vi "Konvolucio MUDS150628 CP1540 Tool.vi"() -> ()   [LabVIEW 2011]
uses:
  <instrlib>/Konvolucio MUDS150628/Types/DtcItemType.ctl
  <vilib>/Utility/miscctls.llb/LVRowAndColumnUnsignedTypeDef.ctl
  <instrlib>/Konvolucio MUDS150628/Types/UdsHandleType.ctl
  <instrlib>/Konvolucio MCAN120803/Types/MCanHandleType.ctl
  <instrlib>/Konvolucio MUDS150628/Public/Low CAN/Attributes/AttrGetPendingMsg.vi
  <instrlib>/Konvolucio MUDS150628/Public/Low CAN/Attributes/AttrGetRxTotal.vi
  <instrlib>/Konvolucio MUDS150628/Public/Low CAN/Attributes/AttrGetRxErrorCounter.vi
  <instrlib>/Konvolucio MUDS150628/Public/Low CAN/Attributes/AttrGetRxDrop.vi
  <instrlib>/Konvolucio MUDS150628/Public/Low CAN/Attributes/AttrGetTxTotal.vi
  <instrlib>/Konvolucio MUDS150628/Public/Low CAN/Attributes/AttrGetTxErrorCounter.vi
  <instrlib>/Konvolucio MUDS150628/Public/Low CAN/Attributes/AttrGetTxDrop.vi
  <instrlib>/Konvolucio MUDS150628/Public/Low CAN/Attributes/AttrSetTermination.vi
  <instrlib>/Konvolucio MUDS150628/Public/Low CAN/Attributes/AttrGetFirmwareRev.vi
  <instrlib>/Konvolucio MUDS150628/Public/Low CAN/Attributes/AttrGetSerialNumber.vi
  <instrlib>/Konvolucio MUDS150628/Public/Low CAN/Attributes/AttrGetAssemblyVersion.vi
  C:/Program Files/National Instruments/LabVIEW 2011/instr.lib/Konvolucio MCAN120803/Private/Konvolucio.MCAN120803.dll
  Konvolucio MCAN120803/Private/Konvolucio.MCAN120803.dll
  <instrlib>/Konvolucio MUDS150628/Konvolucio MUDS150628.lvlib
  <instrlib>/Konvolucio MCAN120803/Konvolucio MCAN120803.lvlib
panel:
  in  "Boolean":bool
  out "Table Control":string[][](table)
  in  "Tab Control 2":enum32{"DTC"}(tab)
  in  "button_DTC_Read":bool
  out "DtcItems":T1[](array[typedef])
  in  "Tab Contorl 3":T2(tab)
  out "TraceibilityValue":string
  in  "button_Tracebility":bool
  in  "button_EEPROM_Request":bool
  out "Request Upload Value":string
  in  "button_LED_IN_GLASS_ADC":bool
  out "LED IN GLASS ADC":u16 format="%04x"
  in  "button_LED_0C42":bool
  in  "button_LED_0C41":bool
  in  "button_LED_0C40":bool
  in  "button_LED_0C39":bool
  in  "Tab Control 1":enum32{"Bus Info"}(tab)
  out "Tx Drop":u32
  out "Tx Error":u32
  out "Tx Total":u32
  out "Rx Drop":u32
  out "Rx Error":u32
  out "Rx Total":u32
  out "Pending Rx":i32
  in  "Tab Control":enum32{"Adapter Info"}(tab)
  out "Fw Revision":string
  out "Serial Number":string
  out "Asm Ver":string
  in  "buttonBusTermination":bool
  in  "button_Pause":bool
  out "indicatorOpen":bool
  in  "button_Stop":bool
  in  "button_Play":bool
  in  "comboAdapters":i32(ring) items=["CAN Bus Adpater - MCAN120803 387536633133 "]
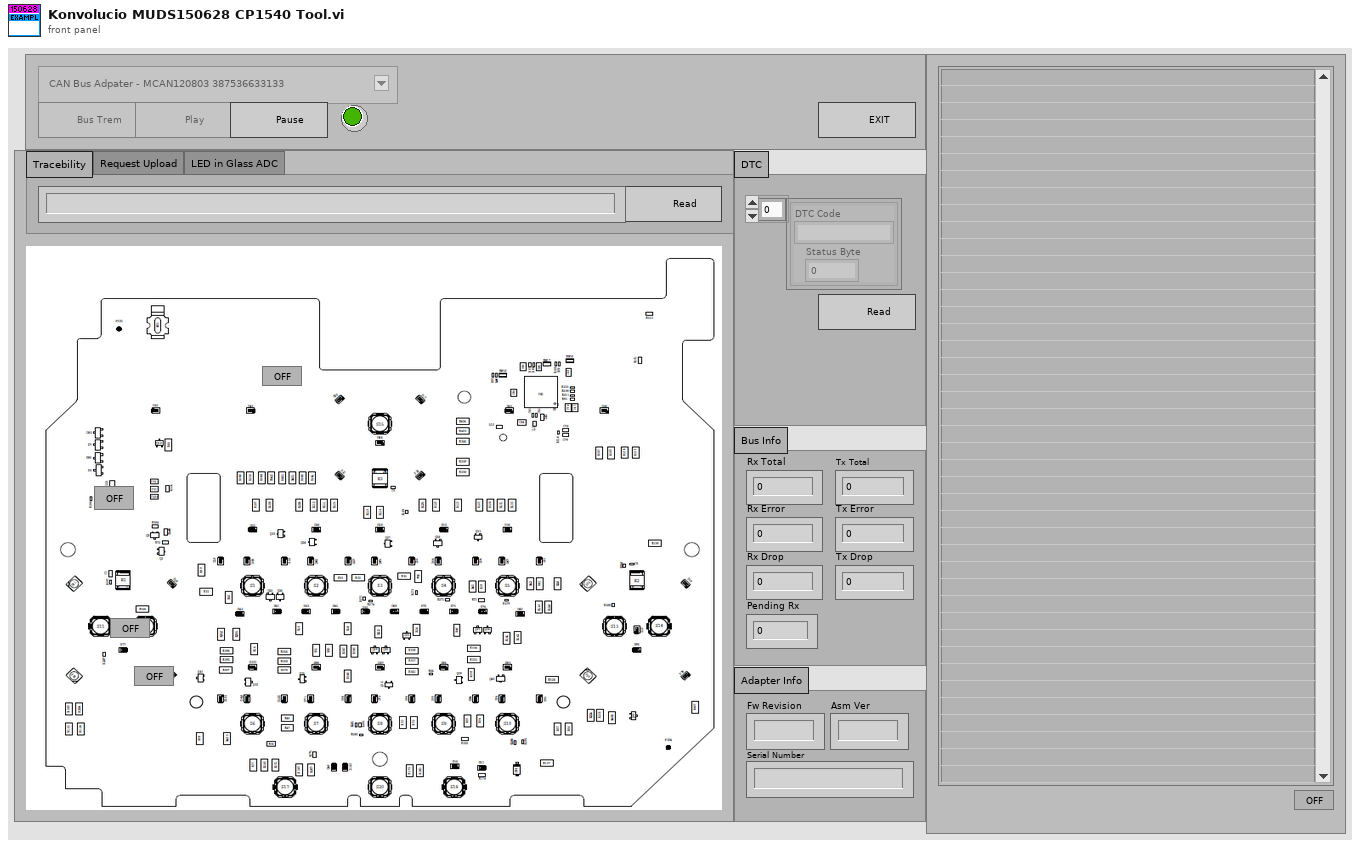
[diagram p1: front panel]
types:
  T1 = typedef "Konvolucio MUDS150628.lvlib/DtcItemType.ctl" = cluster{"DTC Code":string, "Status Byte":i32}
  T2 = enum32{"Tracebility", "Request Upload", "LED in Glass ADC"}
  T3 = typedef "Konvolucio MUDS150628.lvlib/UdsHandleType.ctl" = cluster{"LogPath":path, "LogEnabled":bool, "isOpen":bool, "LogContent":string, "Adapter":string, "MCanHandle":T4, "TransmittId":u32, "ReceiveId":u32}
  T4 = typedef "Konvolucio MCAN120803.lvlib/MCanHandleType.ctl" = cluster{"MCanAdapter":refnum<k24>}
  T5 = typedef "LVRowAndColumnUnsignedTypeDef.ctl" = cluster{"Row":u32, "Column":u32}
  T6 = enum8{"Enabled", "Disabled", "Disabled and Grayed Out"}
  T7 = typedef "Konvolucio MCAN120803.lvlib/AdapterItemType.ctl" = cluster{"Name":string, "DeviceDescription":string, "SerialNumber":string, "InUse":bool, "Handle":refnum<k24>}
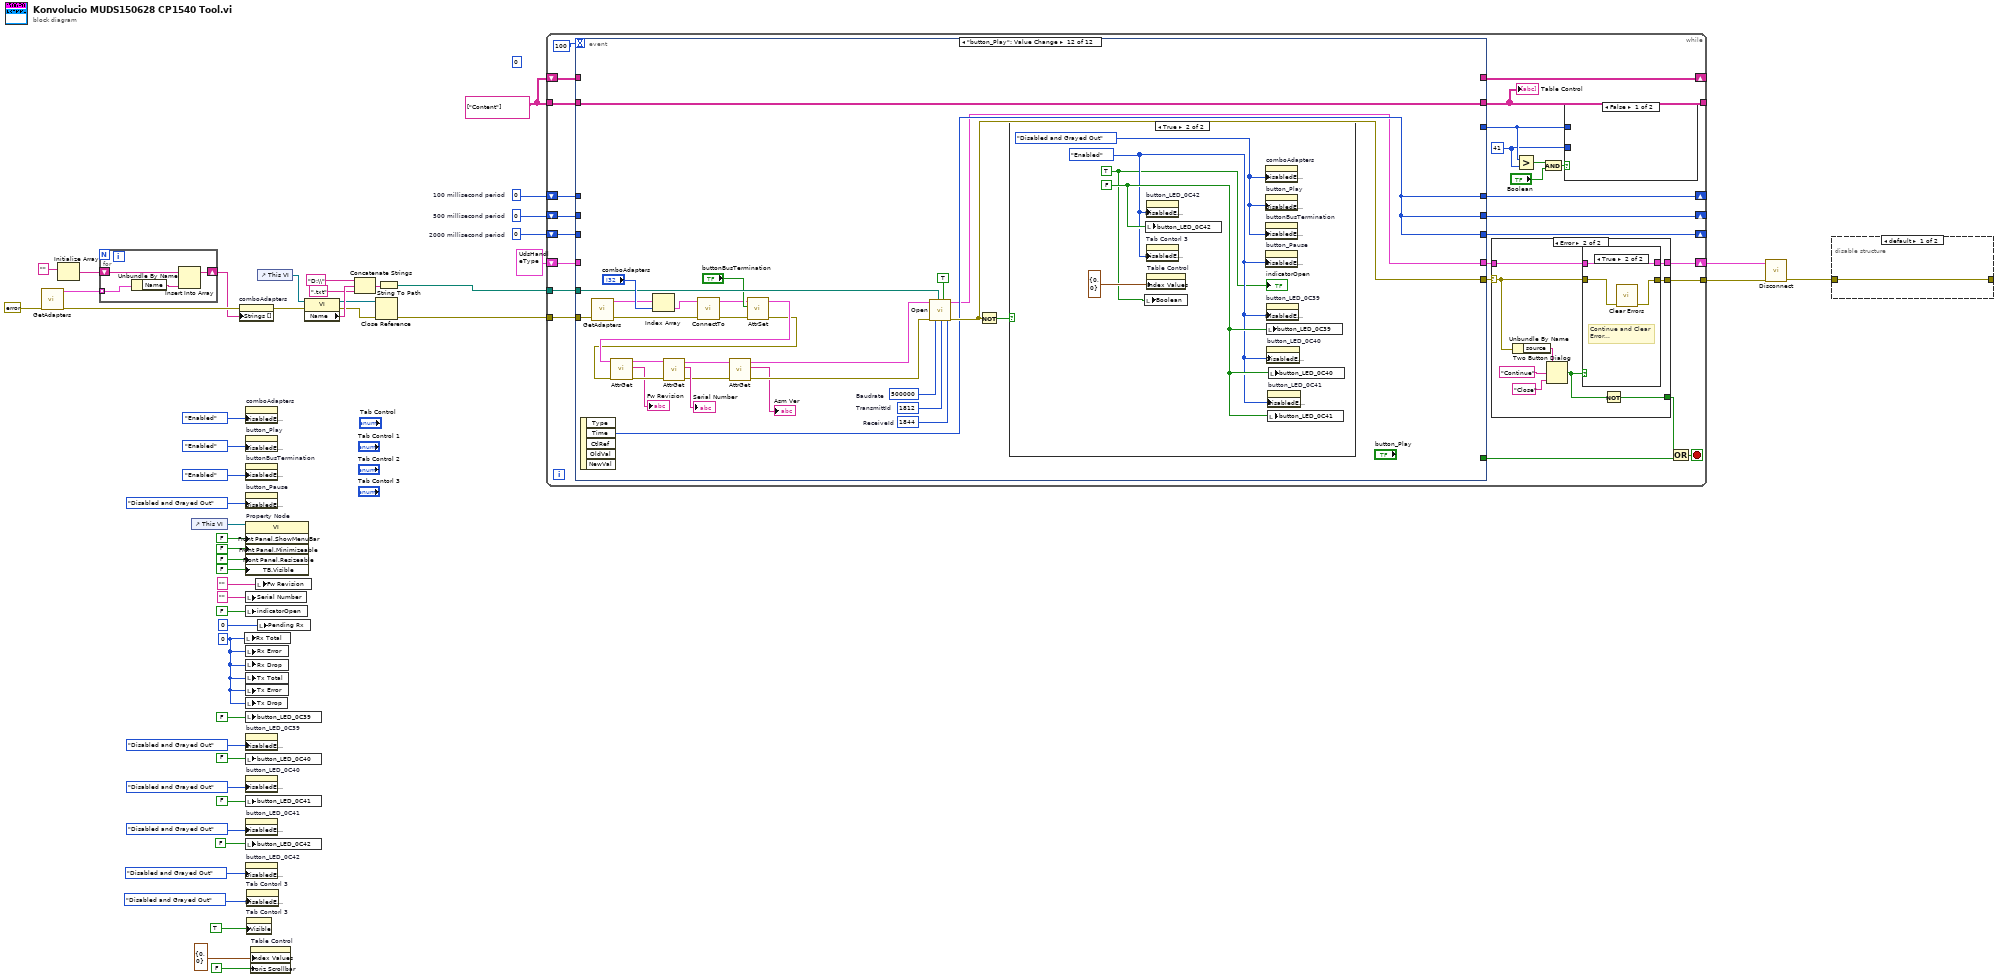
[diagram p0: block diagram]
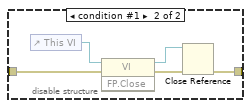
[diagram p2: hidden frame]
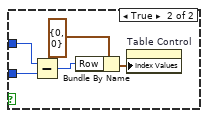
[diagram p3: hidden frame]
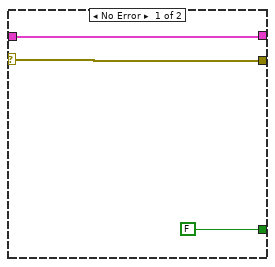
[diagram p4: hidden frame]
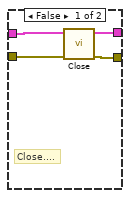
[diagram p5: hidden frame]
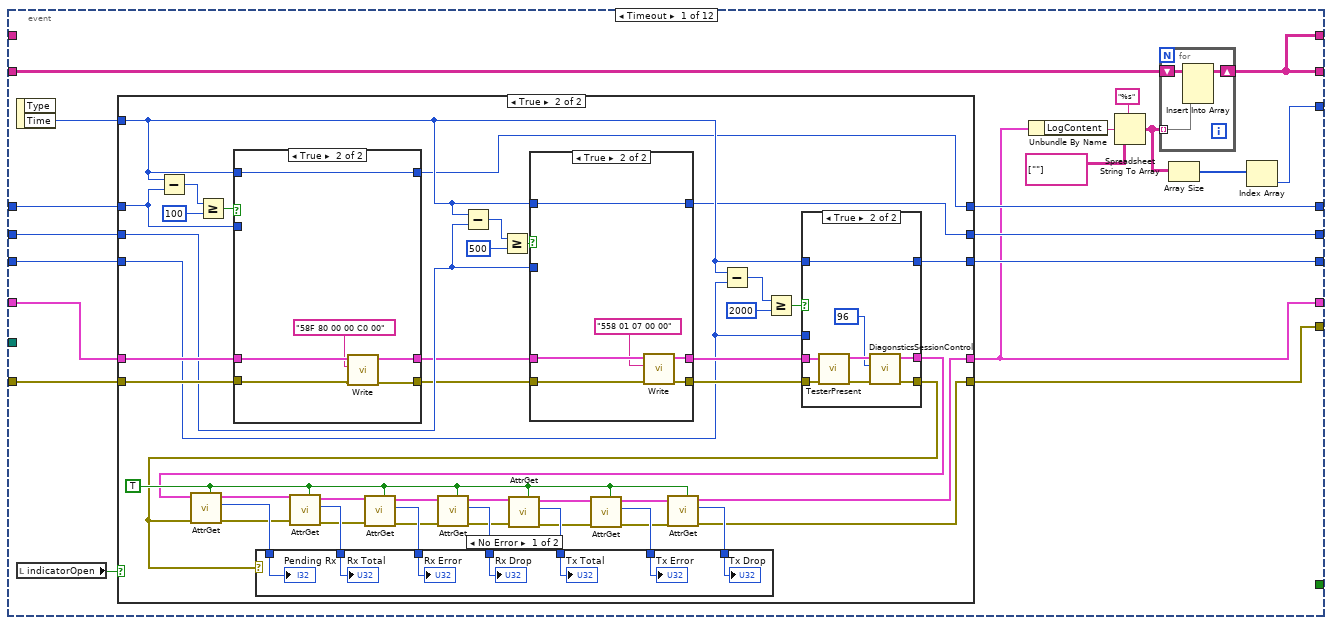
[diagram p6: hidden frame]
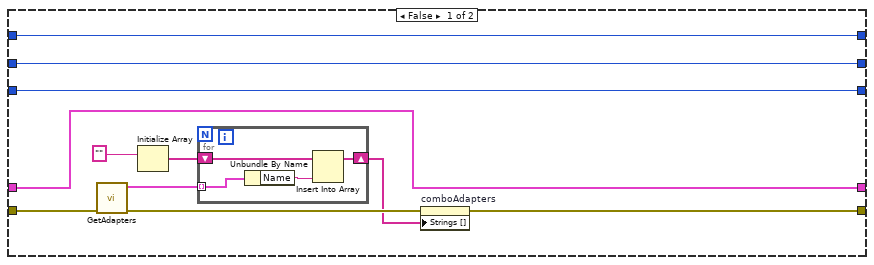
[diagram p7: hidden frame]
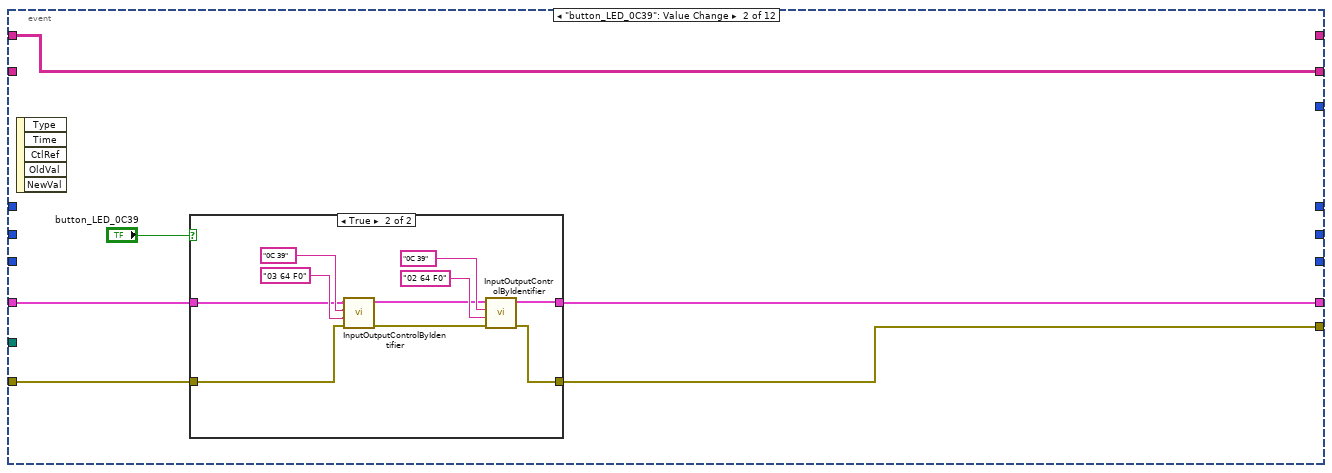
[diagram p12: hidden frame]
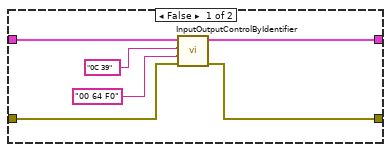
[diagram p13: hidden frame]
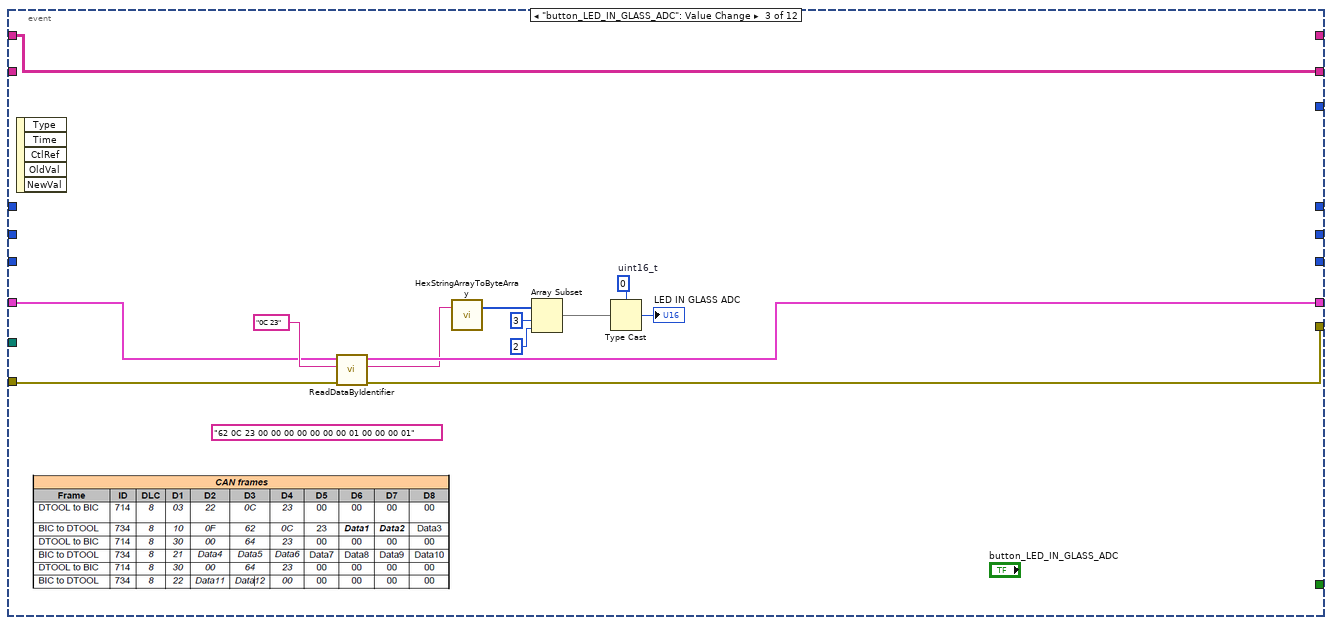
[diagram p14: hidden frame]
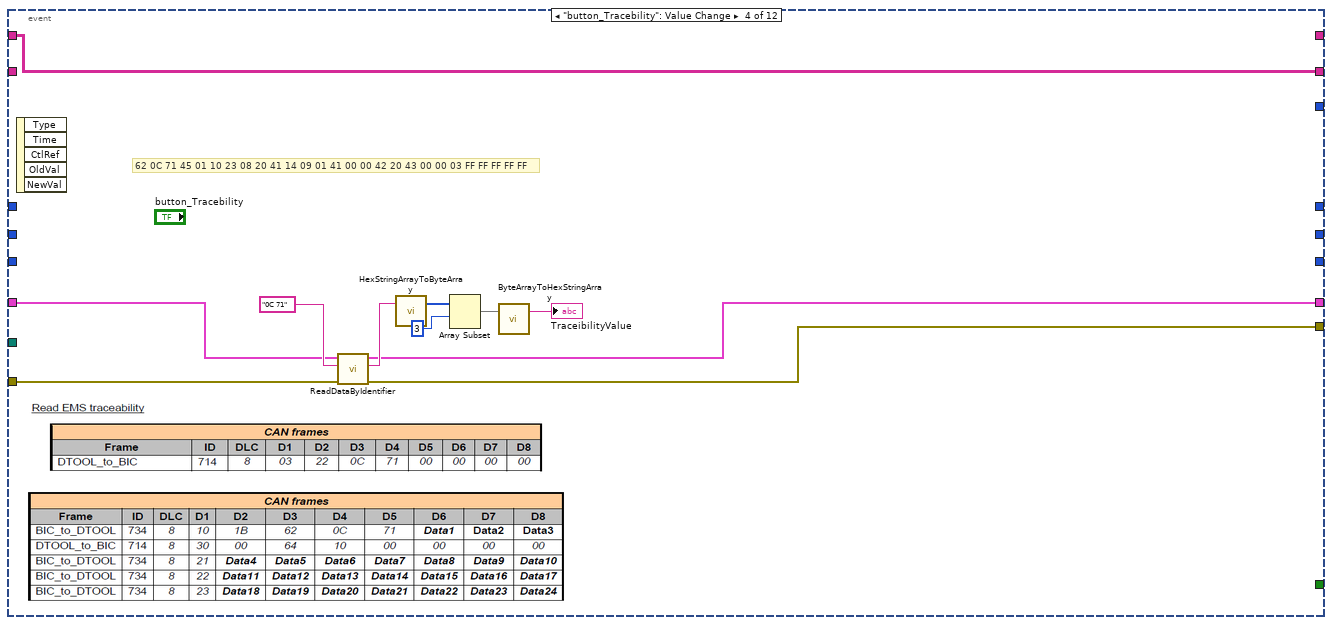
[diagram p15: hidden frame]
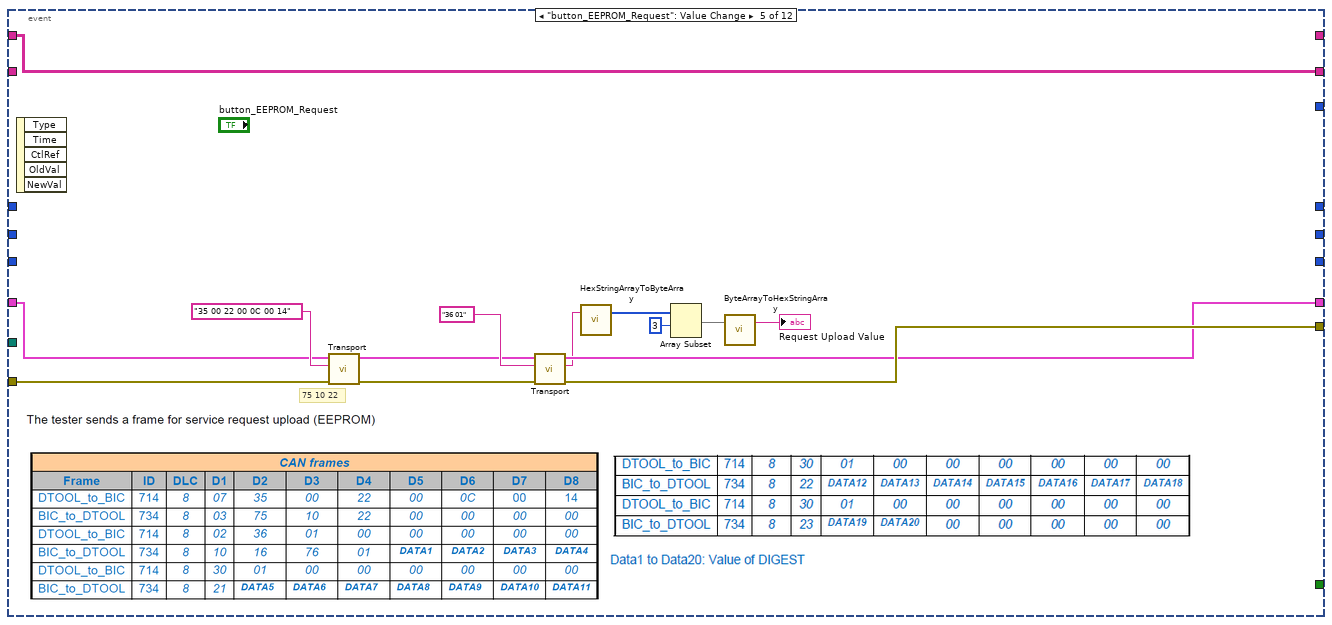
[diagram p16: hidden frame]
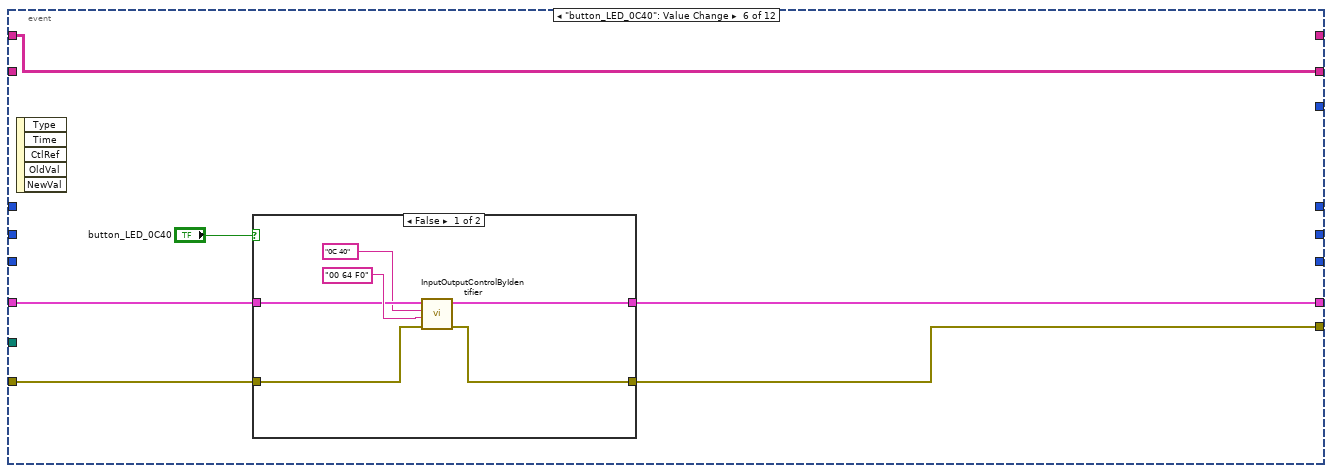
[diagram p17: hidden frame]
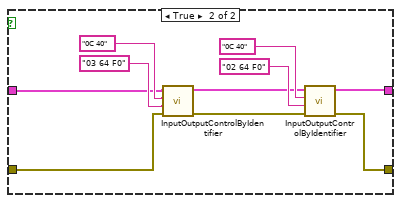
[diagram p18: hidden frame]
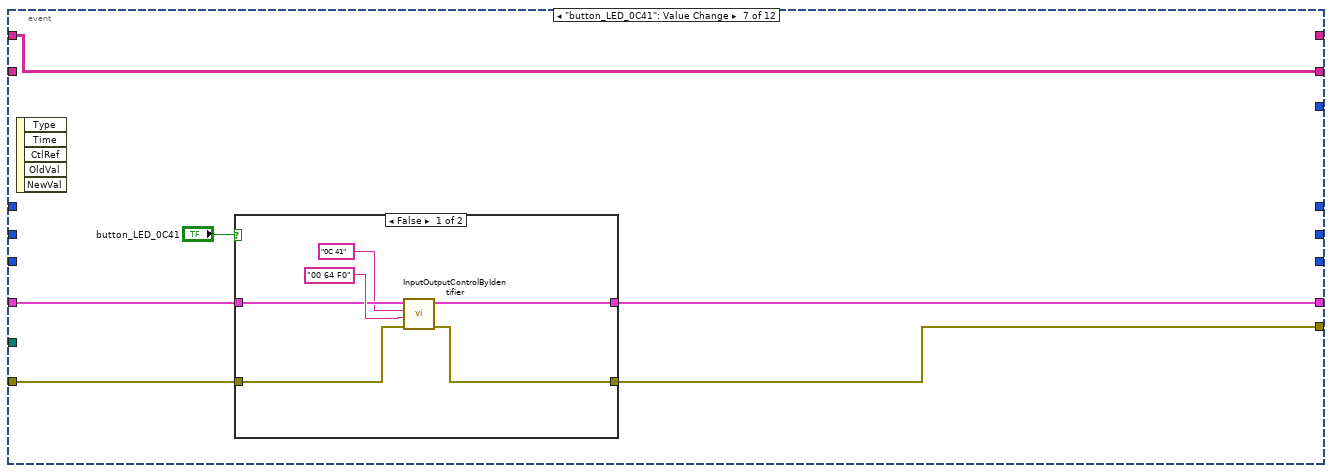
[diagram p19: hidden frame]
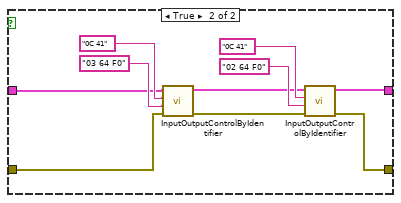
[diagram p20: hidden frame]
diagram:
  (unwired) 0
  w3 = string[][] [["Content"]] ("Table Control 3")
  w16 = u32 0  # 2000 millisecond period
  w17 = u32 0 ("Tx Drop")
  w19 = u32 0  # 500 millisecond period
  w21 = u32 0  # 100 millisecond period
  n1 = call <instrlib>:"GetAdapters.vi"("error in"=errorcluster {"status"=FALSE, "code"=0, "source"=""} ("error in (no error)")) -> ("error out"=w31:errorcluster, "AdaptersOut"=w43:T7[])  [unwired: 9 in]
  n2 = Initialize Array("") -> (w45:string[])  [unwired: 1 in]
  n3 = for {
    tunnel: w43 -> [w52] mode=indexing
    shift-right: [w53] -> w30
    shift-left: w45 -> [w51]
    n4 = Unbundle By Name(w52) -> ("Name"=w54:string)
    n5 = Insert Into Array(array=w51, new element=w54) -> (w53:string[])  [unwired: 1 in]
  }
  n6 = control-ref of="This VI"() -> (w28:refnum<vi>)
  n7 = property on="comboAdapters" class="Ring (strict)"(error in=w31, "Strings []"=w30) -> (error out=w29:errorcluster)  [unwired: 1 in, 1 out]
  n8 = local write "Rx Total"(w17) -> ()
  n9 = property on="comboAdapters" class="Ring (strict)"("DisabledEnum"=T6."Enabled" ("Disabled")) -> ()  [unwired: 2 in, 2 out]
  n10 = property on="button_Play" class="Bool"("DisabledEnum"=T6."Enabled" ("Disabled")) -> ()  [unwired: 2 in, 2 out]
  n11 = property on="buttonBusTermination" class="Bool (strict)"("DisabledEnum"=T6."Enabled" ("Disabled")) -> ()  [unwired: 2 in, 2 out]
  n12 = property on="button_Pause" class="Bool"("DisabledEnum"=T6."Disabled and Grayed Out" ("Disabled")) -> ()  [unwired: 2 in, 2 out]
  n13 = property on="Property Node" class="VI"(reference=w28, "Front Panel.ShowMenuBar"=FALSE ("Front Panel Window:Show Menu Bar"), "Front Panel.Minimizeable"=FALSE ("Front Panel Window:Minimizable"), "Front Panel.Resizeable"=FALSE ("Front Panel Window:Resizable"), "TB.Visible"=FALSE ("Tool Bar:Visible")) -> ()  [unwired: 1 in, 2 out]
  n14 = local write "Serial Number"("" ("Serial Number")) -> ()
  n15 = local write "indicatorOpen"(FALSE ("indicatorOpen")) -> ()
  n16 = local write "Rx Error"(w17) -> ()
  n17 = local write "Rx Drop"(w17) -> ()
  n18 = local write "Tx Total"(w17) -> ()
  n19 = local write "Tx Error"(w17) -> ()
  n20 = local write "Tx Drop"(w17) -> ()
  n21 = local write "button_LED_0C39"(FALSE ("buttonLED_0C39")) -> ()
  n22 = property on="button_LED_0C39" class="Bool (strict)"("DisabledEnum"=T6."Disabled and Grayed Out" ("Disabled")) -> ()  [unwired: 2 in, 2 out]
  n23 = local write "button_LED_0C40"(FALSE ("button_LED_0C40")) -> ()
  n24 = property on="button_LED_0C40" class="Bool (strict)"("DisabledEnum"=T6."Disabled and Grayed Out" ("Disabled")) -> ()  [unwired: 2 in, 2 out]
  n25 = local write "button_LED_0C41"(FALSE ("button_LED_0C41")) -> ()
  n26 = property on="button_LED_0C41" class="Bool (strict)"("DisabledEnum"=T6."Disabled and Grayed Out" ("Disabled")) -> ()  [unwired: 2 in, 2 out]
  n27 = local write "button_LED_0C42"(FALSE ("button_LED_0C42")) -> ()
  n28 = property on="button_LED_0C42" class="Bool (strict)"("DisabledEnum"=T6."Disabled and Grayed Out" ("Disabled")) -> ()  [unwired: 2 in, 2 out]
  n29 = property on="Tab Contorl 3" class="TabCtl (strict)"("DisabledEnum"=T6."Disabled and Grayed Out" ("Disabled")) -> ()  [unwired: 2 in, 2 out]
  n30 = property on="Tab Contorl 3" class="TabCtl (strict)"("Visible"=TRUE) -> ()  [unwired: 2 in, 2 out]
  n31 = property on="Table Control" class="Tbl (strict)"("Index Values"=T5 {"Row"=0, "Column"=0}, "Horiz Scrollbar"=FALSE ("Visible Items:Horizontal Scrollbar Visible")) -> ()  [unwired: 2 in, 2 out]
  n32 = local write "Fw Revision"("" ("Firmware Revision")) -> ()
  n33 = control-ref of="This VI"() -> (w50:refnum<vi>)
  n34 = local write "Pending Rx"(0 ("Pending Messages")) -> ()
  n35 = property class="VI"(reference=w50, error in=w29) -> (reference out=w39:refnum<vi>, error out=w38:errorcluster, "Name"=w48:string)
  n36 = Concatenate Strings("D:\\" ("VI Name"), w48, ".txt" ("string")) -> (w46:string)
  n37 = Close Reference(reference=w39, error in (no error)=w38) -> (error out=w37:errorcluster)
  n38 = String To Path(string=w46) -> (path=w40:path)
  n39 = while {
    tunnel: [w80] -> w42
    tunnel: w37 -> [w75]
    tunnel: w40 -> [w74]
    shift-right: [w72] -> _
    shift-left: w21 -> [w70]
    shift-right: [w68] -> _
    shift-left: w19 -> [w69]
    shift-right: [w66] -> _
    shift-left: w16 -> [w67]
    tunnel: w3 -> [w64]
    tunnel: [w61] -> _
    shift-right: [w63] -> _
    shift-left: w3 -> [w62]
    shift-right: [w55] -> w1
    shift-left: T3 {"LogPath"=path "", "LogEnabled"=FALSE, "isOpen"=FALSE, "LogContent"="", "Adapter"="", "MCanHandle"={"MCanAdapter"=refnum}, "TransmittId"=0, "ReceiveId"=0} ("UdsHandleOut") -> [w71]
    stop <- w79 stop-if-true
    w59 = 41 ("y")
    n40 = event shown="[11] \"button_Play\": Value Change" {
      selector: _ -> [_ _ _ _ _ _ _ _ _ _ _ _]
      dyn-events: _ -> [_ _ _ _ _ _ _ _ _ _ _ _]
      timeout: 100 -> [_ _ _ _ _ _ _ _ _ _ _ _]
      tunnel: [_ _ _ _ _ _ _ "button_Stop" _ _ _ _] -> w77
      tunnel: [w123 w230 w258 w269 w278 w288 w311 w331 w342 w349 w355 w392] -> w76
      tunnel: w75 -> [w122 w229 w259 w270 w284 w289 w312 w331 w343 w352 w358 w398]
      tunnel: [w113 w227 w255 w265 w277 w287 w310 w330 w341 w348 w356 w381] -> w65
      tunnel: w74 -> [_ _ _ _ _ _ _ _ _ _ _ w393]
      tunnel: w70 -> [w120 _ _ _ _ _ _ _ _ _ _ _]
      tunnel: [w119 _ _ _ _ _ _ _ _ _ _ w382] -> w72
      tunnel: w71 -> [w118 w228 w256 w267 w282 w290 w309 w330 w341 w350 w357 _]
      tunnel: w69 -> [w117 _ _ _ _ _ _ _ _ _ _ _]
      tunnel: [w116 _ _ _ _ _ _ _ _ _ _ w382] -> w68
      tunnel: w67 -> [w115 _ _ _ _ _ _ _ _ _ _ _]
      tunnel: [w114 _ _ _ _ _ _ _ _ _ _ w382] -> w66
      tunnel: w64 -> [w109 _ _ _ _ _ _ _ _ _ _ w380]
      tunnel: [w108 w225 w247 w260 w271 w285 w307 w329 w334 w346 w353 w380] -> w61
      tunnel: w62 -> [_ w225 w247 w260 w271 w285 w307 w329 _ w346 w353 _]
      tunnel: [w108 _ _ _ _ _ _ _ w334 _ _ _] -> w63
      tunnel: [w105 _ _ _ _ _ _ _ _ _ _ _] -> w60
      event Timeout {
        n41 = event-data() -> ("Time"=w121:u32)  [unwired: 1 in, 1 out]
        n42 = local read "indicatorOpen"() -> (w124:bool)
        n43 = case shown="True" w124 {
          tunnel: [w132 w156] -> w123
          tunnel: w122 -> [w135 w184]
          tunnel: w121 -> [_ w148]
          tunnel: w120 -> [w131 w185]
          tunnel: [w131 w144] -> w119
          tunnel: w118 -> [w130 w183]
          tunnel: [w130 w155] -> w113
          tunnel: w117 -> [w129 w179]
          tunnel: [w129 w145] -> w116
          tunnel: w115 -> [w128 w146]
          tunnel: [w128 w147] -> w114
          frame False {
            n44 = call <instrlib>:"GetAdapters.vi"("error in"=w135) -> ("error out"=w134:errorcluster, "AdaptersOut"=w136:T7[])  [unwired: 9 in]
            n45 = Initialize Array("") -> (w138:string[])  [unwired: 1 in]
            n46 = for {
              tunnel: w136 -> [w140] mode=indexing
              shift-right: [w141] -> w133
              shift-left: w138 -> [w139]
              n47 = Unbundle By Name(w140) -> ("Name"=w142:string)
              n48 = Insert Into Array(array=w139, new element=w142) -> (w141:string[])  [unwired: 1 in]
            }
            n49 = property on="comboAdapters" class="Ring (strict)"(error in=w134, "Strings []"=w133) -> (error out=w132:errorcluster)  [unwired: 1 in, 1 out]
          }
          frame True {
            w158 = TRUE ("LogSuspend")
            n50 = Subtract(x=w148, y=w185) -> (x-y=w188:u32)
            n51 = Greater Or Equal?(x=w188, y=u32 100) -> (x >= y?=w186:bool)
            n52 = case shown="True" w186 {
              tunnel: w148 -> [_ w224]
              tunnel: [w218 w224] -> w144
              tunnel: w185 -> [w218 _]
              tunnel: w184 -> [w217 w221]
              tunnel: [w217 w220] -> w177
              tunnel: w183 -> [w216 w222]
              tunnel: [w216 w223] -> w178
              frame False {
              }
              frame True {
                n53 = call <instrlib>:"Write.vi"("UdsHandleIn"=w222, "Frame"="58F 80 00 00 C0 00", "error in"=w221) -> ("UdsHandleOut"=w223:T3, "error out"=w220:errorcluster)  [unwired: 6 in]
              }
            }
            n54 = Subtract(x=w148, y=w179) -> (x-y=w182:u32)
            n55 = Greater Or Equal?(x=w182, y=u32 500) -> (x >= y?=w180:bool)
            n56 = case shown="True" w180 {
              tunnel: w148 -> [_ w215]
              tunnel: w179 -> [w207 _]
              tunnel: w178 -> [w209 w212]
              tunnel: w177 -> [w208 w211]
              tunnel: [w209 w213] -> w153
              tunnel: [w208 w214] -> w154
              tunnel: [w207 w215] -> w145
              frame False {
              }
              frame True {
                n57 = call <instrlib>:"Write.vi"("UdsHandleIn"=w212, "Frame"="558 01 07 00 00", "error in"=w211) -> ("UdsHandleOut"=w213:T3, "error out"=w214:errorcluster)  [unwired: 6 in]
              }
            }
            n58 = Subtract(x=w148, y=w146) -> (x-y=w150:u32)
            n59 = Greater Or Equal?(x=w150, y=u32 2000) -> (x >= y?=w151:bool)
            n60 = case shown="True" w151 {
              tunnel: w154 -> [w197 w203]
              tunnel: w153 -> [w198 w202]
              tunnel: [w197 w201] -> w143
              tunnel: [w198 w200] -> w152
              tunnel: w148 -> [_ w199]
              tunnel: [w196 w199] -> w147
              tunnel: w146 -> [w196 _]
              frame False {
              }
              frame True {
                n61 = call <instrlib>:"TesterPresent.vi"("error in"=w203, "UdsHandleIn"=w202) -> ("error out"=w206:errorcluster, "UdsHandleOut"=w205:T3)  [unwired: 8 in]
                n62 = call <instrlib>:"DiagonsticsSessionControl.vi"("error in"=w206, "Session"=u8 96, "UdsHandleIn"=w205) -> ("error out"=w201:errorcluster, "UdsHandleOut"=w200:T3)  [unwired: 7 in]
              }
            }
            n63 = call-poly <instrlib>:"AttrGet.vi"("LogSuspend"=w158, "error in"=w143, "UdsHandleIn"=w152) -> ("error out"=w175:errorcluster, "Value"=w176:i32, "UdsHandleOut"=w174:T3)  [unwired: 6 in]
            n64 = call-poly <instrlib>:"AttrGet.vi"("LogSuspend"=w158, "error in"=w175, "UdsHandleIn"=w174) -> ("error out"=w172:errorcluster, "Value"=w173:u32, "UdsHandleOut"=w171:T3)  [unwired: 6 in]
            n65 = call-poly <instrlib>:"AttrGet.vi"("LogSuspend"=w158, "error in"=w172, "UdsHandleIn"=w171) -> ("error out"=w169:errorcluster, "Value"=w170:u32, "UdsHandleOut"=w168:T3)  [unwired: 6 in]
            n66 = call-poly <instrlib>:"AttrGet.vi"("LogSuspend"=w158, "error in"=w169, "UdsHandleIn"=w168) -> ("error out"=w166:errorcluster, "Value"=w167:u32, "UdsHandleOut"=w165:T3)  [unwired: 6 in]
            n67 = call-poly <instrlib>:"AttrGet.vi"("LogSuspend"=w158, "error in"=w166, "UdsHandleIn"=w165) -> ("error out"=w163:errorcluster, "Value"=w164:u32, "UdsHandleOut"=w162:T3)  [unwired: 6 in]
            n68 = call-poly <instrlib>:"AttrGet.vi"("LogSuspend"=w158, "error in"=w163, "UdsHandleIn"=w162) -> ("error out"=w160:errorcluster, "Value"=w161:u32, "UdsHandleOut"=w159:T3)  [unwired: 6 in]
            n69 = call-poly <instrlib>:"AttrGet.vi"("LogSuspend"=w158, "error in"=w160, "UdsHandleIn"=w159) -> ("error out"=w156:errorcluster, "Value"=w157:u32, "UdsHandleOut"=w155:T3)  [unwired: 6 in]
            n70 = case shown="No Error" w143 {
              tunnel: w176 -> [w195 _]
              tunnel: w173 -> [w194 _]
              tunnel: w170 -> [w193 _]
              tunnel: w167 -> [w192 _]
              tunnel: w164 -> [w191 _]
              tunnel: w161 -> [w190 _]
              tunnel: w157 -> [w189 _]
              frame No Error {
                "Pending Rx" <- w195
                "Rx Total" <- w194
                "Rx Error" <- w193
                "Rx Drop" <- w192
                "Tx Total" <- w191
                "Tx Error" <- w190
                "Tx Drop" <- w189
              }
              frame Error {
              }
            }
          }
        }
        n71 = Unbundle By Name(w113) -> ("LogContent"=w111:string)
        n72 = Spreadsheet String To Array(format string="%s", spreadsheet string=w111, array type (2D Dbl)=string[][] [[""]]) -> (array=w107:string[][])  [unwired: 1 in]
        n73 = for {
          tunnel: w107 -> [w126] mode=indexing
          shift-right: [w125] -> w108
          shift-left: w109 -> [w127]
          n74 = Insert Into Array(array=w127, new element=w126) -> (w125:string[][])  [unwired: 2 in]
        }
        n75 = Array Size(array=w107) -> (size(s)=w106:i32[])
        n76 = Index Array(array=w106) -> (element=w105:i32)  [unwired: 1 in]
      }
      event "button_LED_0C39": Value Change {
        n77 = event-data() -> ()  [unwired: 1 in, 5 out]
        n78 = case shown="True" "button_LED_0C39" {
          tunnel: [w232 w237] -> w230
          tunnel: w229 -> [w231 w246]
          tunnel: w228 -> [w234 w243]
          tunnel: [w233 w238] -> w227
          frame False {
            n79 = call <instrlib>:"InputOutputControlByIdentifier.vi"("error in"=w231, "ControlOption"="00 64 F0" ("DataIn"), "DID"="0C 39", "UdsHandleIn"=w234) -> ("error out"=w232:errorcluster, "UdsHandleOut"=w233:T3)  [unwired: 6 in]
          }
          frame True {
            n80 = call <instrlib>:"InputOutputControlByIdentifier.vi"("error in"=w246, "ControlOption"="03 64 F0" ("DataIn"), "DID"="0C 39", "UdsHandleIn"=w243) -> ("error out"=w240:errorcluster, "UdsHandleOut"=w239:T3)  [unwired: 6 in]
            n81 = call <instrlib>:"InputOutputControlByIdentifier.vi"("error in"=w240, "ControlOption"="02 64 F0" ("DataIn"), "DID"="0C 39", "UdsHandleIn"=w239) -> ("error out"=w237:errorcluster, "UdsHandleOut"=w238:T3)  [unwired: 6 in]
          }
        }
      }
      event "button_LED_IN_GLASS_ADC": Value Change {
        (unwired) "62 0C 23 00 00 00 00 00 00 00 01 00 00 00 01" ("DataOut")
        w252 = u16 0  # uint16_t
        n82 = event-data() -> ()  [unwired: 1 in, 5 out]
        n83 = call <instrlib>:"ReadDataByIdentifier.vi"("error in"=w259, "DID"="0C 23", "UdsHandleIn"=w256) -> ("error out"=w258:errorcluster, "DataOut"=w248:string, "UdsHandleOut"=w255:T3)  [unwired: 6 in]
        n84 = call <instrlib>:"HexStringArrayToByteArray.vi"("HexStirngArray"=w248) -> ("ByteArrayOut"=w249:u8[])  [unwired: 2 in]
        n85 = Array Subset(array=w249, index=3, length=2) -> (w253:u8[])
        n86 = Type Cast(type=w252, x=w253) -> (*(type *) &x=→"LED IN GLASS ADC":u16)
      }
      event "button_Tracebility": Value Change {
        # "62 0C 71 45 01 10 23 08 20 41 14 09 01 41 00 00 42 20 43 00 00 03 FF FF FF FF FF"
        n87 = event-data() -> ()  [unwired: 1 in, 5 out]
        n88 = call <instrlib>:"ReadDataByIdentifier.vi"("error in"=w270, "DID"="0C 71", "UdsHandleIn"=w267) -> ("error out"=w269:errorcluster, "DataOut"=w266:string, "UdsHandleOut"=w265:T3)  [unwired: 6 in]
        n89 = call <instrlib>:"HexStringArrayToByteArray.vi"("HexStirngArray"=w266) -> ("ByteArrayOut"=w263:u8[])  [unwired: 2 in]
        n90 = Array Subset(array=w263, index=3) -> (w262:u8[])  [unwired: 1 in]
        n91 = call <instrlib>:"ByteArrayToHexStringArray.vi"("ByteArrayIn"=w262) -> ("HexStringArrayOut"=→"TraceibilityValue":string)  [unwired: 2 in]
      }
      event "button_EEPROM_Request": Value Change {
        # "75 10 22"
        n92 = event-data() -> ()  [unwired: 1 in, 5 out]
        n93 = call <instrlib>:"Transport.vi"("error in"=w284, "Request"="35 00 22 00 0C 00 14", "UdsHandleIn"=w282) -> ("error out"=w281:errorcluster, "UdsHandleOut"=w279:T3)  [unwired: 6 in, 1 out]
        n94 = call <instrlib>:"Transport.vi"("error in"=w281, "Request"="36 01", "UdsHandleIn"=w279) -> ("error out"=w278:errorcluster, "Response"=w276:string, "UdsHandleOut"=w277:T3)  [unwired: 6 in]
        n95 = call <instrlib>:"HexStringArrayToByteArray.vi"("HexStirngArray"=w276) -> ("ByteArrayOut"=w275:u8[])  [unwired: 2 in]
        n96 = Array Subset(array=w275, index=3) -> (w273:u8[])  [unwired: 1 in]
        n97 = call <instrlib>:"ByteArrayToHexStringArray.vi"("ByteArrayIn"=w273) -> ("HexStringArrayOut"=→"Request Upload Value":string)  [unwired: 2 in]
      }
      event "button_LED_0C40": Value Change {
        n98 = event-data() -> ()  [unwired: 1 in, 5 out]
        n99 = case shown="False" "button_LED_0C40" {
          tunnel: [w293 w298] -> w288
          tunnel: w289 -> [w292 w306]
          tunnel: w290 -> [w295 w303]
          tunnel: [w294 w297] -> w287
          frame False {
            n100 = call <instrlib>:"InputOutputControlByIdentifier.vi"("error in"=w292, "ControlOption"="00 64 F0" ("DataIn"), "DID"="0C 40", "UdsHandleIn"=w295) -> ("error out"=w293:errorcluster, "UdsHandleOut"=w294:T3)  [unwired: 6 in]
          }
          frame True {
            n101 = call <instrlib>:"InputOutputControlByIdentifier.vi"("error in"=w306, "ControlOption"="03 64 F0" ("DataIn"), "DID"="0C 40", "UdsHandleIn"=w303) -> ("error out"=w300:errorcluster, "UdsHandleOut"=w299:T3)  [unwired: 6 in]
            n102 = call <instrlib>:"InputOutputControlByIdentifier.vi"("error in"=w300, "ControlOption"="02 64 F0" ("DataIn"), "DID"="0C 40", "UdsHandleIn"=w299) -> ("error out"=w298:errorcluster, "UdsHandleOut"=w297:T3)  [unwired: 6 in]
          }
        }
      }
      event "button_LED_0C41": Value Change {
        n103 = event-data() -> ()  [unwired: 1 in, 5 out]
        n104 = case shown="False" "button_LED_0C41" {
          tunnel: [w315 w320] -> w311
          tunnel: w312 -> [w314 w328]
          tunnel: w309 -> [w317 w325]
          tunnel: [w316 w319] -> w310
          frame False {
            n105 = call <instrlib>:"InputOutputControlByIdentifier.vi"("error in"=w314, "ControlOption"="00 64 F0" ("DataIn"), "DID"="0C 41", "UdsHandleIn"=w317) -> ("error out"=w315:errorcluster, "UdsHandleOut"=w316:T3)  [unwired: 6 in]
          }
          frame True {
            n106 = call <instrlib>:"InputOutputControlByIdentifier.vi"("error in"=w328, "ControlOption"="03 64 F0" ("DataIn"), "DID"="0C 41", "UdsHandleIn"=w325) -> ("error out"=w322:errorcluster, "UdsHandleOut"=w321:T3)  [unwired: 6 in]
            n107 = call <instrlib>:"InputOutputControlByIdentifier.vi"("error in"=w322, "ControlOption"="02 64 F0" ("DataIn"), "DID"="0C 41", "UdsHandleIn"=w321) -> ("error out"=w320:errorcluster, "UdsHandleOut"=w319:T3)  [unwired: 6 in]
          }
        }
      }
      event "button_Stop": Value Change {
        n108 = event-data() -> ()  [unwired: 1 in, 5 out]
      }
      event "button_Pause": Value Change {
        w334 = string[][] [["Content"]] ("Table Control 3")
        w338 = u32 0 ("Pending Messages")
        w336 = FALSE ("indicatorOpen")
        w337 = T6."Enabled" ("Disabled")
        w335 = T6."Disabled and Grayed Out" ("Disabled")
        n109 = event-data() -> ()  [unwired: 1 in, 5 out]
        n110 = call <instrlib>:"Close.vi"("error in"=w343, "UdsHandleIn"=w341) -> ("error out"=w345:errorcluster, "UdsHandleOut"=w344:T3)  [unwired: 8 in]
        n111 = call <instrlib>:"Disconnect.vi"("error in"=w345, "UdsHandleIn"=w344) -> ("error out"=w342:errorcluster)  [unwired: 9 in]
        n112 = property on="button_LED_0C40" class="Bool (strict)"("DisabledEnum"=w335) -> ()  [unwired: 2 in, 2 out]
        n113 = local write "button_LED_0C41"(w336) -> ()
        n114 = property on="button_LED_0C41" class="Bool (strict)"("DisabledEnum"=w335) -> ()  [unwired: 2 in, 2 out]
        n115 = local write "button_LED_0C42"(w336) -> ()
        n116 = property on="button_LED_0C42" class="Bool (strict)"("DisabledEnum"=w335) -> ()  [unwired: 2 in, 2 out]
        n117 = property on="Tab Contorl 3" class="TabCtl (strict)"("DisabledEnum"=w335) -> ()  [unwired: 2 in, 2 out]
        n118 = local write "Boolean"(FALSE ("Boolean")) -> ()
        n119 = local write "Rx Total"(w338) -> ()
        n120 = property on="comboAdapters" class="Ring (strict)"("DisabledEnum"=w337) -> ()  [unwired: 2 in, 2 out]
        n121 = property on="button_Play" class="Bool"("DisabledEnum"=w337) -> ()  [unwired: 2 in, 2 out]
        n122 = property on="buttonBusTermination" class="Bool (strict)"("DisabledEnum"=w337) -> ()  [unwired: 2 in, 2 out]
        n123 = property on="button_Pause" class="Bool"("DisabledEnum"=w335) -> ()  [unwired: 2 in, 2 out]
        n124 = local write "Serial Number"("") -> ()
        n125 = local write "indicatorOpen"(w336) -> ()
        n126 = local write "Rx Error"(w338) -> ()
        n127 = local write "Rx Drop"(w338) -> ()
        n128 = local write "Tx Total"(w338) -> ()
        n129 = local write "Tx Error"(w338) -> ()
        n130 = local write "Tx Drop"(w338) -> ()
        n131 = local write "button_LED_0C39"(w336) -> ()
        n132 = property on="button_LED_0C39" class="Bool (strict)"("DisabledEnum"=w335) -> ()  [unwired: 2 in, 2 out]
        n133 = local write "button_LED_0C40"(w336) -> ()
        n134 = local write "Fw Revision"("") -> ()
        n135 = local write "Pending Rx"(w338) -> ()
      }
      event "button_DTC_Read": Value Change {
        n136 = event-data() -> ()  [unwired: 1 in, 5 out]
        n137 = call <instrlib>:"ReadDtc.vi"("error in"=w352, "Paramter"="02 29", "UdsHandleIn"=w350) -> ("error out"=w349:errorcluster, "DtcItems"=→"DtcItems":T1[], "UdsHandleOut"=w348:T3)  [unwired: 5 in, 1 out]
      }
      event "button_LED_0C42": Value Change {
        n138 = event-data() -> ()  [unwired: 1 in, 5 out]
        n139 = case shown="False" "button_LED_0C42" {
          tunnel: [w361 w366] -> w355
          tunnel: w358 -> [w360 w374]
          tunnel: w357 -> [w363 w371]
          tunnel: [w362 w365] -> w356
          frame False {
            n140 = call <instrlib>:"InputOutputControlByIdentifier.vi"("error in"=w360, "ControlOption"="00 64 F0" ("DataIn"), "DID"="0C 42", "UdsHandleIn"=w363) -> ("error out"=w361:errorcluster, "UdsHandleOut"=w362:T3)  [unwired: 6 in]
          }
          frame True {
            n141 = call <instrlib>:"InputOutputControlByIdentifier.vi"("error in"=w374, "ControlOption"="03 64 F0" ("DataIn"), "DID"="0C 42", "UdsHandleIn"=w371) -> ("error out"=w368:errorcluster, "UdsHandleOut"=w367:T3)  [unwired: 6 in]
            n142 = call <instrlib>:"InputOutputControlByIdentifier.vi"("error in"=w368, "ControlOption"="02 64 F0" ("DataIn"), "DID"="0C 42", "UdsHandleIn"=w367) -> ("error out"=w366:errorcluster, "UdsHandleOut"=w365:T3)  [unwired: 6 in]
          }
        }
      }
      event "button_Play": Value Change {
        w401 = u32 500000  # Baudrate
        w403 = u32 1844  # ReceiveId
        w402 = u32 1812  # TransmittId
        n143 = event-data() -> ("Time"=w382:u32)  [unwired: 1 in, 4 out]
        n144 = call <instrlib>:"GetAdapters.vi"("error in"=w398) -> ("error out"=w396:errorcluster, "AdaptersOut"=w397:T7[])  [unwired: 9 in]
        n145 = Index Array(array=w397, index="comboAdapters") -> (element=w395:T7)
        n146 = call <instrlib>:"ConnectTo.vi"("error in"=w396, "AdapterIn"=w395) -> ("error out"=w390:errorcluster, "UdsHandleOut"=w389:T3)  [unwired: 8 in]
        n147 = call-poly <instrlib>:"AttrSet.vi"("error in"=w390, "Enabled"="buttonBusTermination", "UdsHandleIn"=w389) -> ("error out"=w387:errorcluster, "UdsHandleOut"=w388:T3)  [unwired: 7 in]
        n148 = call-poly <instrlib>:"AttrGet.vi"("error in"=w387, "UdsHandleIn"=w388) -> ("error out"=w385:errorcluster, "Value"=→"Fw Revision":string, "UdsHandleOut"=w386:T3)  [unwired: 7 in]
        n149 = call-poly <instrlib>:"AttrGet.vi"("error in"=w385, "UdsHandleIn"=w386) -> ("error out"=w379:errorcluster, "Value"=→"Serial Number":string, "UdsHandleOut"=w378:T3)  [unwired: 7 in]
        n150 = call-poly <instrlib>:"AttrGet.vi"("error in"=w379, "UdsHandleIn"=w378) -> ("error out"=w377:errorcluster, "Value"=→"Asm Ver":string, "UdsHandleOut"=w376:T3)  [unwired: 7 in]
        n151 = call <instrlib>:"Open.vi"("ReceiveId"=w403, "LogEnabled"=TRUE, "TransmittId"=w402, "LogPath"=w393, "error in"=w377, "BaudRate"=w401, "UdsHandleIn"=w376) -> ("error out"=w392:errorcluster, "UdsHandleOut"=w381:T3)  [unwired: 3 in]
        n152 = Not(x=w392) -> (.not. x?=w394:bool)
        n153 = case shown="True" w394 {
          frame False {
          }
          frame True {
            w407 = FALSE ("button_LED_0C39")
            w404 = TRUE ("indicatorOpen")
            w406 = T6."Enabled" ("Disabled")
            w408 = T6."Disabled and Grayed Out" ("Disabled")
            n154 = local write "Boolean"(w404) -> ()
            n155 = local write "button_LED_0C42"(w407) -> ()
            n156 = property on="button_LED_0C42" class="Bool (strict)"("DisabledEnum"=w406) -> ()  [unwired: 2 in, 2 out]
            n157 = property on="Tab Contorl 3" class="TabCtl (strict)"("DisabledEnum"=w406) -> ()  [unwired: 2 in, 2 out]
            n158 = property on="Table Control" class="Tbl (strict)"("Index Values"=T5 {"Row"=0, "Column"=0}) -> ()  [unwired: 2 in, 2 out]
            n159 = property on="comboAdapters" class="Ring (strict)"("DisabledEnum"=w408) -> ()  [unwired: 2 in, 2 out]
            n160 = property on="button_Play" class="Bool"("DisabledEnum"=w408) -> ()  [unwired: 2 in, 2 out]
            n161 = property on="buttonBusTermination" class="Bool (strict)"("DisabledEnum"=w408) -> ()  [unwired: 2 in, 2 out]
            n162 = property on="button_Pause" class="Bool"("DisabledEnum"=w406) -> ()  [unwired: 2 in, 2 out]
            n163 = property on="button_LED_0C39" class="Bool (strict)"("DisabledEnum"=w406) -> ()  [unwired: 2 in, 2 out]
            n164 = local write "button_LED_0C39"(w407) -> ()
            n165 = property on="button_LED_0C40" class="Bool (strict)"("DisabledEnum"=w406) -> ()  [unwired: 2 in, 2 out]
            n166 = property on="button_LED_0C41" class="Bool (strict)"("DisabledEnum"=w406) -> ()  [unwired: 2 in, 2 out]
            n167 = local write "button_LED_0C41"(w407) -> ()
            n168 = local write "button_LED_0C40"(w407) -> ()
            "indicatorOpen" <- w404
          }
        }
      }
    }
    "Table Control" <- w61
    n169 = case shown="Error" w76 {
      selector: w76 -> [w88 w94]
      tunnel: [w88 w93] -> w80
      tunnel: [FALSE w91] -> w78
      tunnel: [w86 w90] -> w55
      tunnel: w65 -> [w86 w89]
      frame No Error {
      }
      frame Error {
        n170 = Unbundle By Name(w94) -> ("source"=w97:string)
        n171 = Two Button Dialog(message=w97, 1:"Close" ("F button name (\"Cancel\")"), 2:"Continue" ("T button name (\"OK\")")) -> (T button?=w92:bool)
        n172 = case shown="True" w92 {
          tunnel: w94 -> [w98 w102]
          tunnel: [w101 w104] -> w93
          tunnel: [w100 w103] -> w90
          tunnel: w89 -> [w99 w103]
          frame False {
            # "Close...."
            n173 = call <instrlib>:"Close.vi"("error in"=w98, "UdsHandleIn"=w99) -> ("error out"=w101:errorcluster, "UdsHandleOut"=w100:T3)  [unwired: 8 in]
          }
          frame True {
            # "Continue and Clear\nError..."
            n174 = call <vilib>:"Clear Errors.vi"("error in (no error)"=w102) -> ("error out"=w104:errorcluster)  [unwired: 6 in]
          }
        }
        n175 = Not(x=w92) -> (.not. x?=w91:bool)
      }
    }
    n176 = Greater?(x=w60, y=w59) -> (0:w57:bool)
    n177 = And(x=w57, y="Boolean") -> (x .and. y?=w58:bool)
    n178 = case shown="False" w58 {
      tunnel: w59 -> [_ w81]
      tunnel: w60 -> [_ w82]
      frame False {
      }
      frame True {
        n179 = Subtract(x=w82, y=w81) -> (x-y=w83:i32)
        n180 = Bundle By Name(cluster=T5 {"Row"=0, "Column"=0} ("Index Values"), "Row"=w83) -> (w84:T5)
        n181 = property on="Table Control" class="Tbl (strict)"("Index Values"=w84) -> ()  [unwired: 2 in, 2 out]
      }
    }
    n182 = Or(x=w78, y=w77) -> (x .or. y?=w79:bool)
  }
  n183 = call <instrlib>:"Disconnect.vi"("error in"=w42, "UdsHandleIn"=w1) -> ("error out"=w41:errorcluster)  [unwired: 9 in]
  n184 = disable-structure shown="default" {
    disable-tunnel: w41 -> [w409 w411]
    disable-tunnel: [w409 w410] -> _
    frame condition #0 (active) {
    }
    frame condition #1 {
      n185 = control-ref of="This VI"() -> (w413:refnum<vi>)
      n186 = invoke class="VI" method="FP.Close"(reference=w413, error in=w411) -> (reference out=w412:refnum<vi>, error out=w414:errorcluster)  [unwired: 1 in, 1 out]
      n187 = Close Reference(reference=w412, error in (no error)=w414) -> (error out=w410:errorcluster)
    }
  }
